vi "DAQ_E_mIO_DIO.destructor.vi"(0 "i ref in":refnum<vi>, 5 "error in (no error)":errorcluster) -> (19 "error out":errorcluster)   [LabVIEW 2014, in "DAQ_E_mIO_DIO.lvlib"]
doc: "This is the destructor of a class.\n\nLicense Agreement for this software:\n\nCopyright (C)\nGesellschaft für Schwerionenforschung, GSI\nPlanckstr. 1\n64291 Darmstadt\nGermany\n\nContact: D.Beck@gsi.de \n\nThis program is free software; you can redistribute it and/or modify it under the terms of the \nGNU General Public License as published by the Free Software Foundation; either version 2 of \nthe license, or (at your option) any later version.\n\nThis program is distributed in the hope that it will be useful, but WITHOUT ANY WARRANTY; \nwithout even the implied warranty of MERCHANTABILITY or FITNESS FOR A PARTICULAR PURPOSE. See the GNU General License for more details (http://www.gnu.org).\n\nGesellschaft für Schwerionenforschung, GSI\nPlanckstr. 1, 64291 Darmstadt, Germany\nFor all questions and ideas contact: M.Richter@gsi.de, H.Brand@gsi.de or D.Beck@gsi.de.\nLast update: 16-JUN-2004"
uses:
  DAQ_E_mIO_DIO.lvlib
  CS_Core/CSApplicationBaseClasses/DigiIOBase/DigiIOBase.lvlib
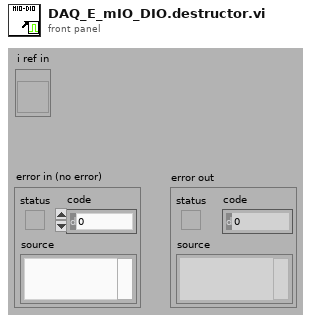
[diagram p1: front panel]
types:
  T1 = typedef "DAQ_E_mIO_DIO.lvlib/DAQ_E_mIO_DIO.i attribute.ctl" = cluster{"DOutChannel":refnum<k21>, "DInChannel":refnum<k21>, "nOfBitsIn":i32, "nOfBitsOut":i32}
  T2 = enum16{"SetAttribute", "GetAttribute", "CreateAttribute", "DestroyAttribute", "DestroyAllAtributes"}
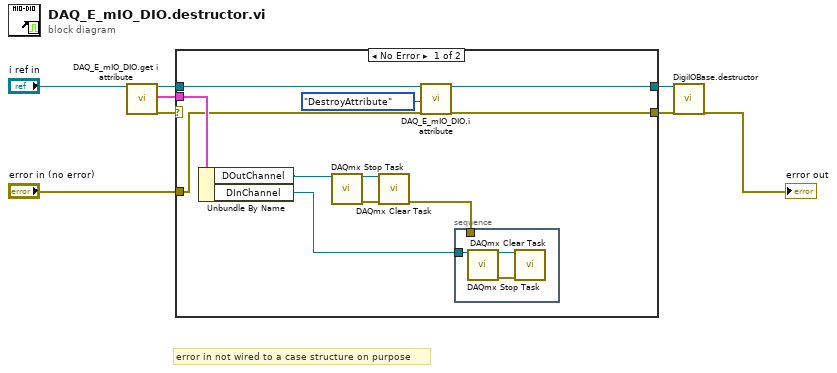
[diagram p0: block diagram]
diagram:
  # "error in not wired to a case structure on purpose"
  n1 = call "DAQ_E_mIO_DIO.get i attribute.vi"("i ref in"="i ref in") -> ("i ref out"=w4:refnum<vi>, "i attribute"=w3:T1, "error out"=w2:errorcluster)  [unwired: 16 in]
  n2 = case shown="No Error" w2 {
    tunnel: [w18 w24] -> w8
    tunnel: [w17 w23] -> w7
    tunnel: w4 -> [w16 w24]
    tunnel: w3 -> [w15 _]
    tunnel: "error in (no error)" -> [w9 w23]
    frame No Error {
      n3 = Unbundle By Name(w15) -> ("DOutChannel"=w12:refnum<k21>, "DInChannel"=w11:refnum<k21>)
      n4 = call <vilib>:"DAQmx Stop Task.vi"("task/channels in"=w12) -> ("task out"=w13:refnum<k21>, "error out"=w14:errorcluster)  [unwired: 13 in]
      n5 = call <vilib>:"DAQmx Clear Task.vi"("task in"=w13, "error in"=w14) -> ("error out"=w10:errorcluster)  [unwired: 13 in]
      n6 = call "DAQ_E_mIO_DIO.i attribute.vi"("VI Refnum"=w16, "Action"=T2."DestroyAttribute", "error in (no error)"=w9) -> ("VI Refnum out"=w18:refnum<vi>, "error out"=w17:errorcluster)  [unwired: 14 in, 1 out]
      n7 = stacked-sequence {
        tunnel: w11 -> [w21]
        tunnel: w10 -> [_]
        frame #0 {
          n8 = call <vilib>:"DAQmx Stop Task.vi"("task/channels in"=w21) -> ("task out"=w20:refnum<k21>, "error out"=w22:errorcluster)  [unwired: 13 in]
          n9 = call <vilib>:"DAQmx Clear Task.vi"("task in"=w20, "error in"=w22) -> ()  [unwired: 13 in, 1 out]
        }
      }
    }
    frame Error {
    }
  }
  n10 = call "DigiIOBase.destructor.vi"("i ref in"=w8, "error in (no error)"=w7) -> ("error out"=→"error out":errorcluster)  [unwired: 17 in]
